vi "SubVI of linear equation.vi"(1 "X":dbl, 2 "B":dbl, 3 "A":dbl) -> (0 "Numeric":dbl)   [LabVIEW 2009]
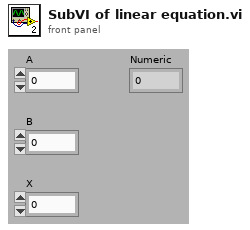
[diagram p1: front panel]
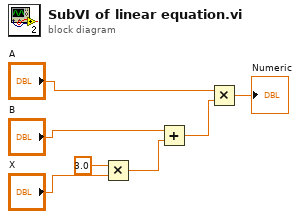
[diagram p0: block diagram]
diagram:
  n1 = Multiply(x=3.0, y="X") -> (x*y=w4:dbl)
  n2 = Add(x="B", y=w4) -> (x+y=w5:dbl)
  n3 = Multiply(x="A", y=w5) -> (x*y=→"Numeric":dbl)
